vi "AprilTag Target Package Vers 2.vi"(0 "Camera Name":string="cam0") -> ()   [LabVIEW 2023]
uses:
  <vilib>/vision/Image Controls.llb/IMAQ Image.ctl
  <vilib>/Utility/config.llb/NI_LVConfig.lvlib
  <vilib>/Utility/config.llb/Write Key (String).vi
  Camera Set Up/Event Setup Types.ctl
  <vilib>/vision/NI_Vision_Development_Module.lvlib
  <vilib>/Rock Robotics/Network Tables/NT Write Numeric Array.vi
  <vilib>/Utility/config.llb/Read Key (String).vi
  <vilib>/vision/Pattern Matching.llb/IMAQ Match Range Setting.ctl
  <vilib>/vision/Shape Detection.llb/ShapeDetectionMatchOptions.ctl
  <vilib>/Rock Robotics/Network Tables/NT Write Integer Array.vi
panel:
  in  "Main":enum32{"Page 1", "Page 2"}(tab)
  out "Image":T1(plugin-control)
  in  "Settings":bool
  in  "Save":bool
  in  "Tools":bool
  out "Fps":dbl format="%#.0f"
  in  "Target Size":dbl=6.5
  out "Distance":dbl[](array[numeric]) format="%.1f"
  out "Angle":dbl[](array[numeric]) format="%.1f"
  in  "Find Tag Number":bool
  in  "Min Score":dbl=800.0
  in  "Min Rect Size (pix)":dbl
  in  "Max Rect Size (pix)":dbl
  in  "Home":bool
  in  "upper limit":sgl=1.2
  in  "lower limit":sgl=0.8
  # "Aspect Ratio"
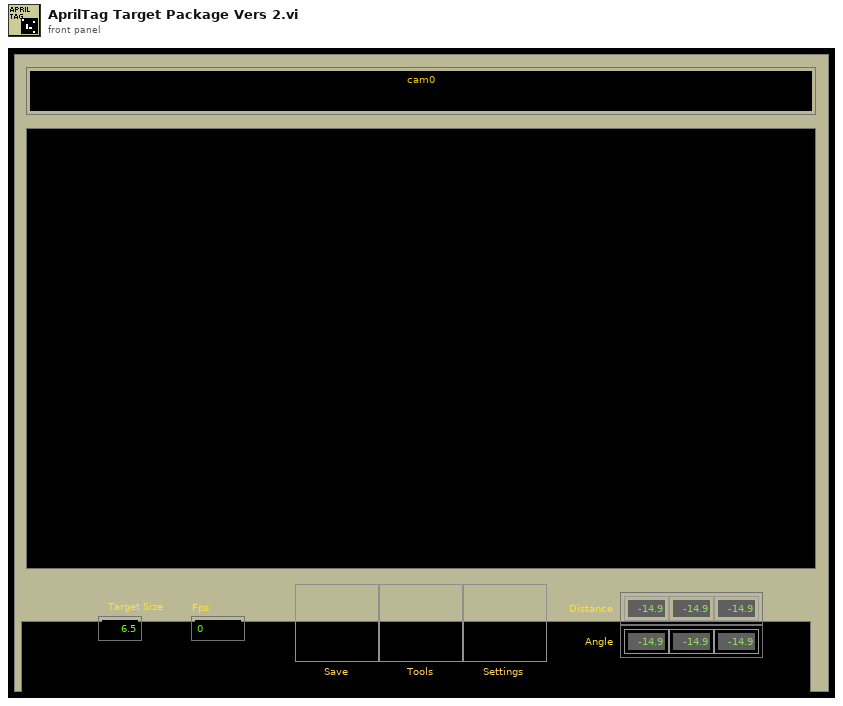
[diagram p1: front panel]
types:
  T1 = typedef "IMAQ Image.ctl" = refnum<image>
  T2 = typedef "Image Type" = u32
  T3 = typedef "ShapeDetectionMatchOptions.ctl" = cluster{"Rotation":bool, "Scale":bool, "Occlusion":bool, "Range Settings":T4[]}
  T4 = typedef "IMAQ Match Range Setting.ctl" = cluster{"Match Constraints":u32, "Min":dbl, "Max":dbl}
  T5 = cluster{"Min Width":dbl, "Max Width":dbl, "Min Height":dbl, "Max Height":dbl}
  T6 = typedef "Event Setup Types.ctl" = enum16{"Default", "Camera Loop Started", "Close Settings", "GreyScale", "Open Front Panel", "Save Data", "Exit"}
  T7 = cluster{"Corners":cluster{"X":sgl, "Y":sgl}[], "Angle":dbl, "Width":dbl, "Height":dbl, "Score":dbl}[]
  T8 = typedef "AprilTag Target Fields.ctl" = cluster{"diameter points":cluster{"first point":cluster{"x":dbl, "y":dbl}, "projected point":cluster{"x":dbl, "y":dbl}}, "normalized center":cluster{"x":dbl, "y":dbl}, "Overall Score":dbl, "Distance (ft)":dbl, "Offset Angle":dbl, "Tag corner points":cluster{"X":dbl, "Y":dbl}[], "Tag Center":cluster{"X":dbl, "Y":dbl}, "Tag Yaw":dbl, "Tag Pitch":dbl, "AprilTag Number":i32}
  T9 = typedef "Target Fields.ctl" = cluster{"diameter points":cluster{"first point":cluster{"x":dbl, "y":dbl}, "projected point":cluster{"x":dbl, "y":dbl}}, "normalized center":cluster{"x":dbl, "y":dbl}, "Overall Score":dbl, "Area Score":dbl, "Moment Score":dbl, "Aspect Score":dbl, "Distance (ft)":dbl, "Upper Goal":bool}
  T10 = typedef "NI_LVConfig.lvlib/Config Data RefNum.ctl" = refnum<k1>
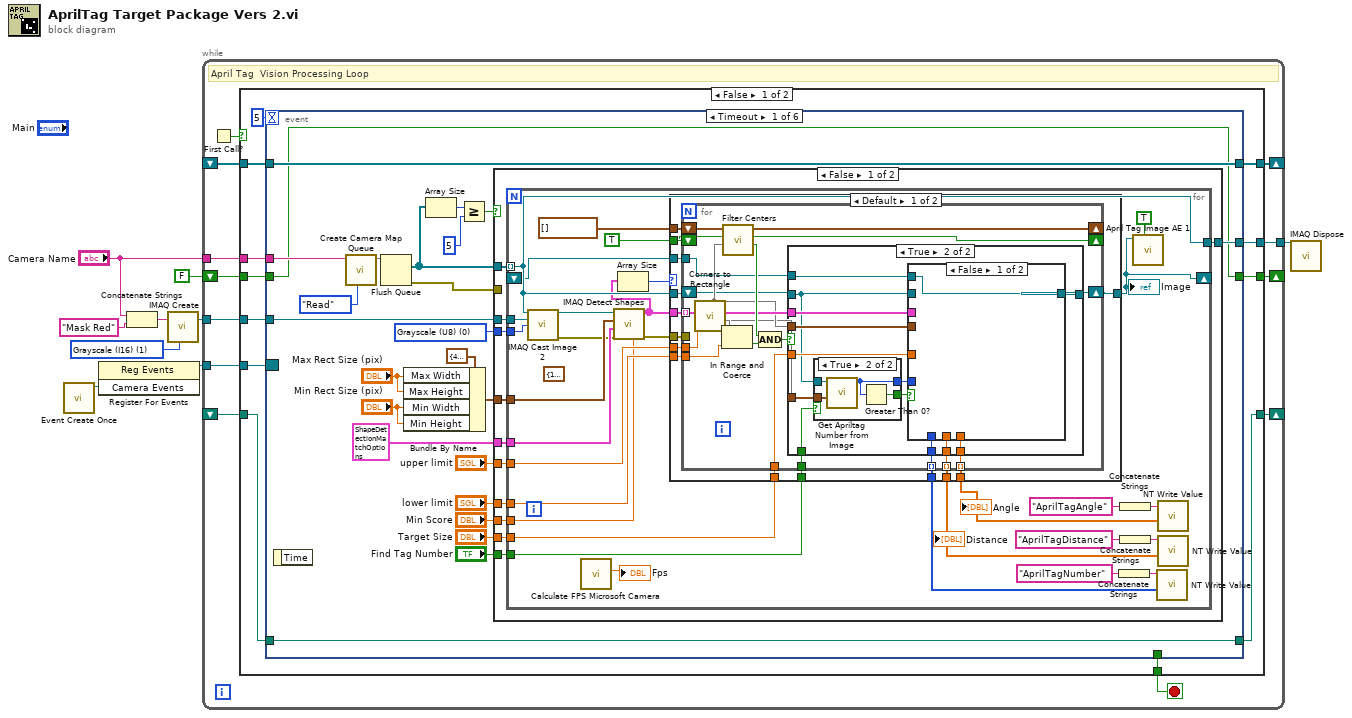
[diagram p0: block diagram]
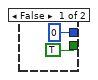
[diagram p3: hidden frame]
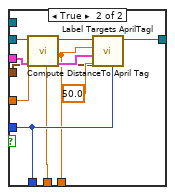
[diagram p4: hidden frame]
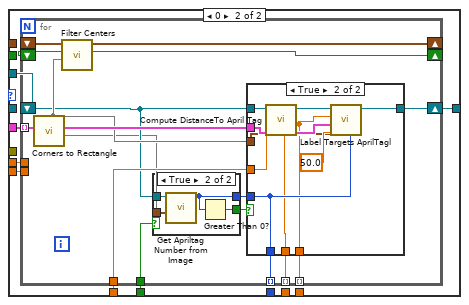
[diagram p5: hidden frame]
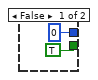
[diagram p6: hidden frame]
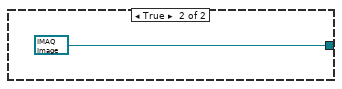
[diagram p8: hidden frame]
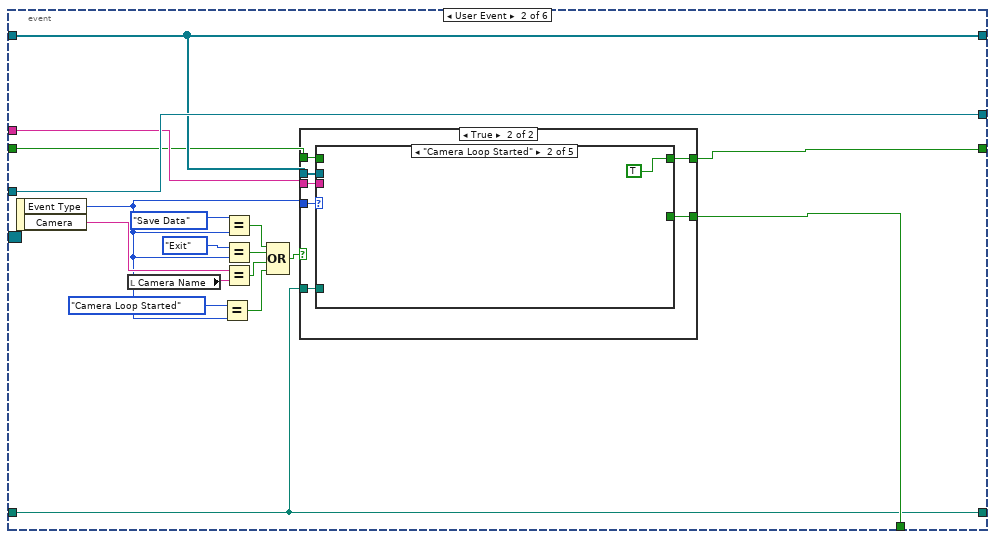
[diagram p9: hidden frame]
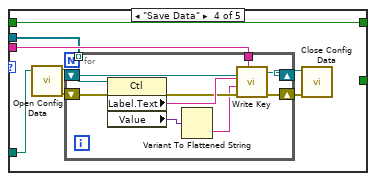
[diagram p13: hidden frame]
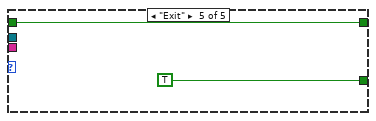
[diagram p14: hidden frame]
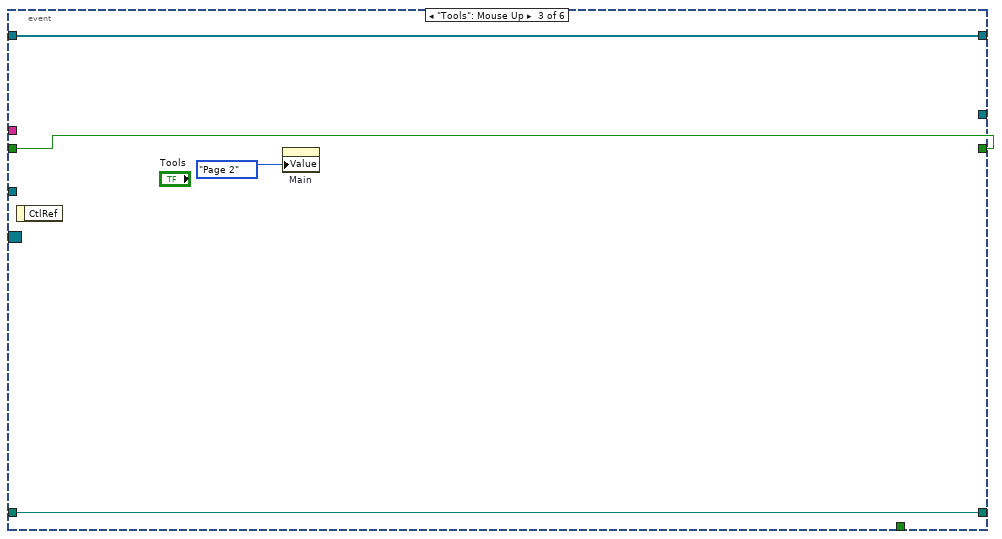
[diagram p15: hidden frame]
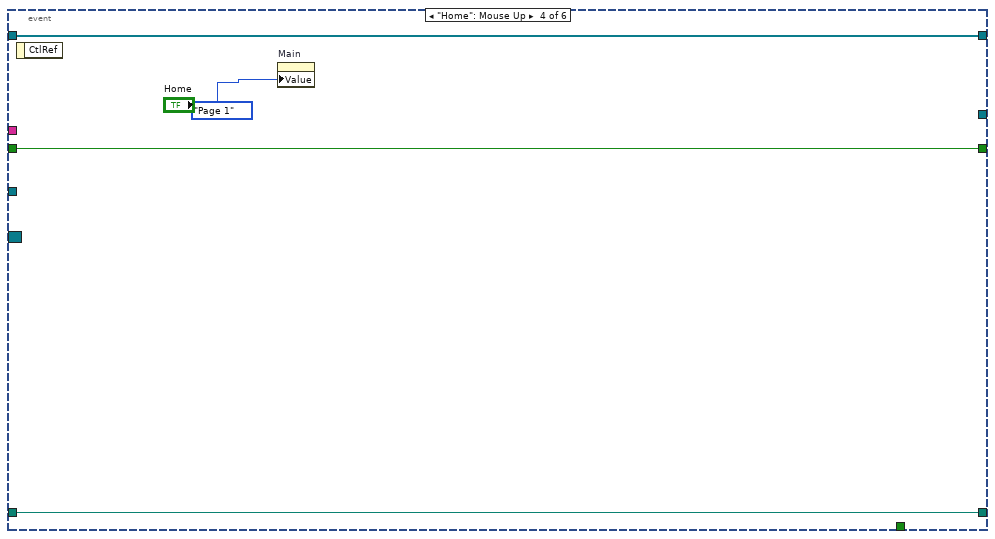
[diagram p16: hidden frame]
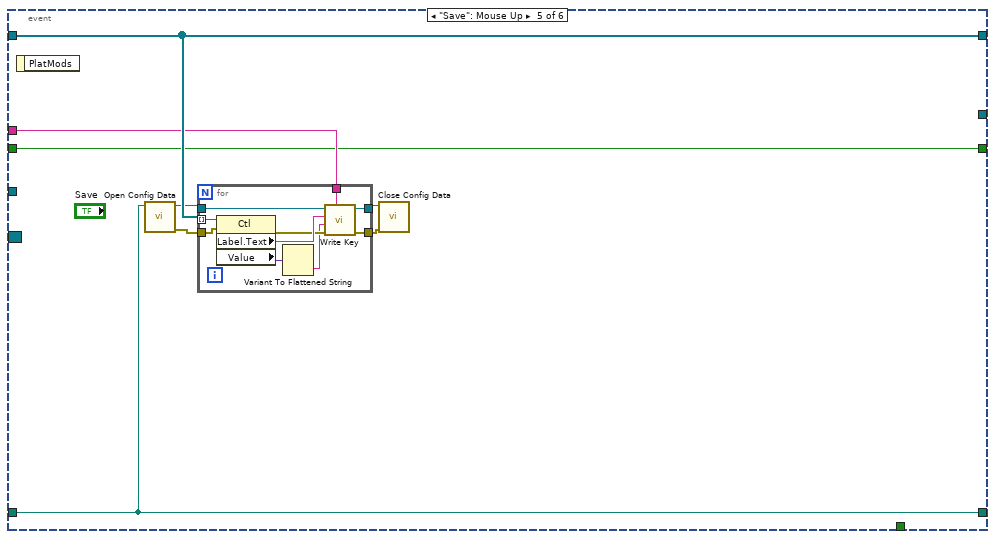
[diagram p17: hidden frame]
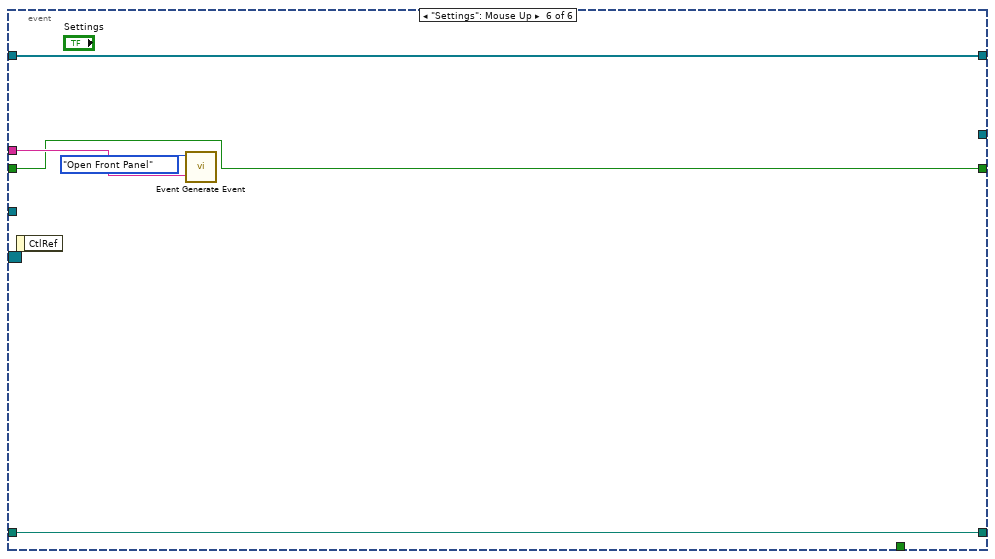
[diagram p18: hidden frame]
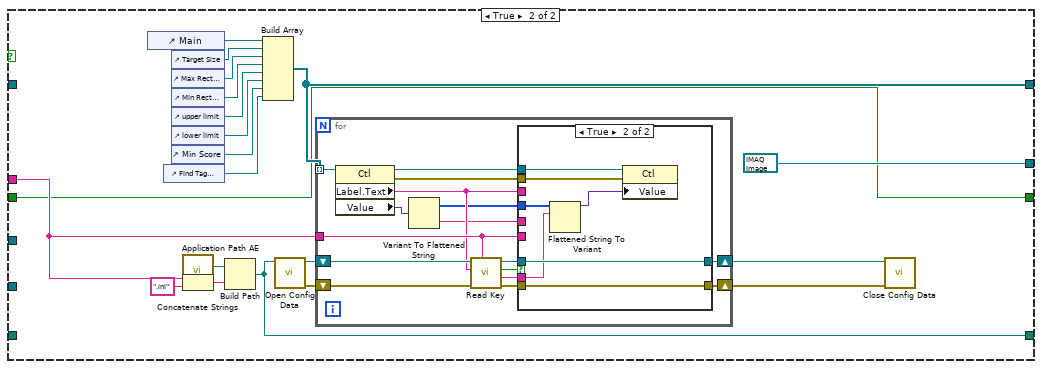
[diagram p19: hidden frame]
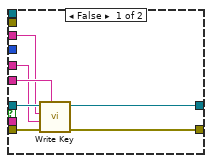
[diagram p20: hidden frame]
diagram:
  w6 = T2 1 items=["Grayscale (U8)", "Grayscale (I16)", "Grayscale (SGL)", "Complex (CSG)", "RGB (U32)", "HSL (U32)", "RGB (U64)", "Grayscale (U16)"] ("Image Type")
  n1 = call "Event Create Once.vi"() -> ("Camera Events"=w8:refnum<user-event>)  [unwired: 10 in, 1 out]
  n2 = register-events(w8) -> (reference out=w7:refnum<event-registration>)  [unwired: 2 in, 1 out]
  n3 = Concatenate Strings("Camera Name", "Mask Red" ("string")) -> (w5:string)
  n4 = call "IMAQ Create"("Image Name"=w5, "Image Type"=w6) -> ("New Image"=w9:T1)  [unwired: 2 in, 2 out]
  n5 = while {
    tunnel: w9 -> [w21]
    tunnel: [w20] -> w1
    tunnel: w7 -> [w19]
    tunnel: "Camera Name" -> [w17]
    shift-right: [w15] -> _
    shift-left: _ -> [w14]
    shift-right: [w13] -> _
    shift-left: _ -> [w12]
    shift-right: [w10] -> _
    shift-left: FALSE -> [w11]
    stop <- w18 stop-if-true
    # "April Tag  Vision Processing Loop"
    n6 = First Call?() -> (First Call?: T/F=w16:bool)
    n7 = case shown="False" w16 {
      tunnel: w21 -> [w33 _]
      tunnel: [w32 T1 refnum ("New Image")] -> w20
      tunnel: w19 -> [w31 _]
      tunnel: [w30 _] -> w18
      tunnel: w17 -> [w29 w303]
      tunnel: [w27 w299] -> w15
      tunnel: w14 -> [w28 _]
      tunnel: [w26 w302] -> w13
      tunnel: w12 -> [w24 _]
      tunnel: w11 -> [w23 w296]
      tunnel: [w22 w296] -> w10
      frame False {
        n8 = event shown="[0] Timeout" {
          selector: w31 -> [_ _ _ _ _ _]
          dyn-events: _ -> [_ _ _ _ _ _]
          timeout: 5 -> [_ _ _ _ _ _]
          tunnel: w33 -> [w56 w227 _ _ _ _]
          tunnel: [w57 w227 _ _ _ _] -> w32
          tunnel: [_ w226 _ _ _ _] -> w30
          tunnel: w29 -> [w53 w225 _ _ w270 w286]
          tunnel: w28 -> [w55 w223 w262 w266 w273 w289]
          tunnel: [w55 w223 w262 w266 w273 w289] -> w27
          tunnel: w24 -> [w54 w224 w261 w265 w274 w288]
          tunnel: [w54 w224 w261 w265 w274 w288] -> w26
          tunnel: w23 -> [w52 w214 w259 w263 w267 w285]
          tunnel: [w52 w213 w259 w263 w267 w285] -> w22
          event Timeout {
            w47 = T2 0 items=["Grayscale (U8)", "Grayscale (I16)", "Grayscale (SGL)", "Complex (CSG)", "RGB (U32)", "HSL (U32)", "RGB (U64)", "Grayscale (U16)"] ("Image Type")
            n9 = event-data() -> ()  [unwired: 1 in, 1 out]
            n10 = call "Create Camera Map Queue.vi"("Action"=enum16{"Read", "Write"}."Read", "Camera"=w53) -> (3:w49)  [unwired: 7 in, 2 out]
            n11 = Flush Queue(queue=w49) -> (remaining elements=w34:T1[], error out=w48:errorcluster)  [unwired: 1 in, 1 out]
            n12 = Bundle By Name(cluster=T5 {"Min Width"=40.0, "Max Width"=100.0, "Min Height"=40.0, "Max Height"=200.0} ("Rectangle Descriptor"), "Max Width"="Max Rect Size (pix)", "Max Height"="Max Rect Size (pix)", "Min Width"="Min Rect Size (pix)", "Min Height"="Min Rect Size (pix)") -> (w41:T5)
            n13 = Array Size(array=w34) -> (size(s)=w46:i32)
            n14 = Greater Or Equal?(x=w46, y=5) -> (x >= y?=w44:bool)
            n15 = case shown="False" w44 {
              tunnel: [w62 T1 refnum ("Image")] -> w57
              tunnel: w56 -> [w68 _]
              tunnel: "Target Size" -> [w67 _]
              tunnel: w34 -> [w66 _]
              tunnel: w48 -> [_ _]
              tunnel: w47 -> [w65 _]
              tunnel: w41 -> [w64 _]
              tunnel: T3 {"Rotation"=TRUE, "Scale"=TRUE, "Occlusion"=FALSE, "Range Settings"=[{"Match Constraints"=0, "Min"=-25.0, "Max"=25.0}, {"Match Constraints"=1, "Min"=25.0, "Max"=150.0}, {"Match Constraints"=0, "Min"=-25.0, "Max"=25.0}]} ("Match Options") -> [w63 _]
              tunnel: "lower limit" -> [w61 _]
              tunnel: "upper limit" -> [w60 _]
              tunnel: "Min Score" -> [w59 _]
              tunnel: "Find Tag Number" -> [w58 _]
              frame False {
                n16 = for {
                  tunnel: w68 -> [w98]
                  tunnel: w66 -> [w80] mode=indexing
                  tunnel: w67 -> [w91]
                  tunnel: w65 -> [w97]
                  tunnel: w64 -> [w95]
                  tunnel: w63 -> [w94]
                  tunnel: [w80] -> w62
                  tunnel: w61 -> [w89]
                  tunnel: w60 -> [w88]
                  tunnel: w59 -> [w79]
                  tunnel: w58 -> [w73]
                  shift-right: [w70] -> _
                  shift-left: _ -> [w69]
                  (unwired) cluster{"Lower value":sgl, "Upper value":sgl} {"Lower value"=128.0, "Upper value"=255.0} ("Range")
                  n17 = call "IMAQ Cast Image 2"("Image Src"=w80, "Image Dst"=w98, "Image Type"=w97) -> ("Image Dst Out"=w74:T1, "error out"=w78:errorcluster)  [unwired: 11 in]
                  n18 = call "Calculate FPS Microsoft Camera.vi"() -> ("Fps"=→"Fps":dbl)  [unwired: 11 in]
                  n19 = call-poly "IMAQ Detect Shapes"("Minimum match score"=w79, "error in (no error)"=w78, "Match Options"=w94, "Rectangle Descriptor"=w95, "Image"=w74) -> ("error out"=w90:errorcluster, "Rectangles"=w72:T7)  [unwired: 4 in, 1 out]
                  n20 = Array Size(array=w72) -> (size(s)=w71:i32)
                  n21 = case shown="Default" w71 {
                    tunnel: cluster{"X":dbl, "Y":dbl}[] [] ("Centers 2") -> [w112 _]
                    tunnel: TRUE -> [w111 _]
                    tunnel: w72 -> [w110 w173]
                    tunnel: w91 -> [w109 w172]
                    tunnel: w90 -> [w108 _]
                    tunnel: w89 -> [w107 w169]
                    tunnel: w88 -> [w106 w170]
                    tunnel: [w105 _] -> w84
                    tunnel: [w104 _] -> w82
                    tunnel: [w103 w168] -> w70
                    tunnel: w80 -> [w102 _]
                    tunnel: [w101 _] -> w75
                    tunnel: w73 -> [w100 w171]
                    tunnel: w69 -> [w99 w167]
                    frame Default {
                      n22 = for {
                        shift-right: [w120] -> w103
                        shift-left: w102 -> [w118]
                        shift-right: [w132] -> _
                        shift-left: w112 -> [w133]
                        shift-right: [w130] -> _
                        shift-left: w111 -> [w131]
                        tunnel: w110 -> [w116] mode=indexing
                        tunnel: w109 -> [w125]
                        tunnel: [w124] -> w104 mode=indexing
                        tunnel: [w123] -> w105 mode=indexing
                        tunnel: w108 -> [_]
                        tunnel: w107 -> [w122]
                        tunnel: w106 -> [w121]
                        tunnel: [w115] -> w101 mode=indexing
                        tunnel: w100 -> [w114]
                        tunnel: w99 -> [w113]
                        n23 = call "Corners to Rectangle.vi"("tag info"=w116) -> ("output cluster"=w126:T8, 4:w134, 5:w119, 6:w117)  [unwired: 7 in]
                        n24 = In Range and Coerce(upper limit=w121, x=w134, lower limit=w122) -> (In Range?=w128:bool)  [unwired: 1 out]
                        n25 = call "Filter Centers.vi"("Center"=w119, "First time"=w131, "Centers"=w133) -> ("Added"=w129:bool, "First time Out"=w130:bool, "Centers 2"=w132:cluster{"X":dbl, "Y":dbl}[])  [unwired: 6 in]
                        n26 = Compound Arithmetic op=AND(w129, w128) -> (w127:bool)
                        n27 = case shown="True" w127 {
                          tunnel: w118 -> [_ w141]
                          tunnel: [w135 w148] -> w120
                          tunnel: w126 -> [_ w147]
                          tunnel: w125 -> [_ w146]
                          tunnel: [_ w145] -> w124
                          tunnel: [_ w144] -> w123
                          tunnel: w119 -> [_ w143]
                          tunnel: w117 -> [_ w142]
                          tunnel: [_ w139] -> w115
                          tunnel: w114 -> [_ w137]
                          tunnel: w113 -> [w135 w136]
                          frame False {
                          }
                          frame True {
                            n28 = case shown="True" w137 {
                              tunnel: w142 -> [_ w154]
                              tunnel: w141 -> [_ w153]
                              tunnel: [0 ("AprilTag#") w152] -> w140
                              tunnel: [TRUE w151] -> w138
                              frame False {
                              }
                              frame True {
                                n29 = call "Get Apriltag Number from Image.vi"("Corners"=w154, "Image"=w153) -> ("AprilTag#"=w152:i32)  [unwired: 9 in]
                                n30 = Greater Than 0?(x=w152) -> (x > 0?=w151:bool)
                              }
                            }
                            n31 = case shown="False" w138 {
                              tunnel: [w155 w166] -> w148
                              tunnel: w147 -> [_ w163]
                              tunnel: w146 -> [_ w162]
                              tunnel: [_ w156] -> w145
                              tunnel: [_ w157] -> w144
                              tunnel: w143 -> [_ w160]
                              tunnel: w141 -> [_ w159]
                              tunnel: w140 -> [_ w158]
                              tunnel: [_ w158] -> w139
                              tunnel: w136 -> [w155 _]
                              frame False {
                              }
                              frame True {
                                n32 = call "Compute DistanceTo April Tag.vi"("Target Width (in)"=w162, "results"=w163, "Image Src"=w159) -> ("results out"=w164:T9, "Off Angle"=w157:dbl, "Image Dst Out"=w161:T1, "Distance"=w156:dbl)  [unwired: 4 in, 1 out]
                                n33 = call "Label Targets AprilTagl.vi"(4:w158, 6:w160, 8:50.0 ("Score Threshold"), "results"=w164, "Angle"=w157, "Image in"=w161) -> ("Image out"=w166:T1)  [unwired: 5 in]
                              }
                            }
                          }
                        }
                      }
                    }
                    frame 0 {
                      n34 = for {
                        shift-right: [w182] -> w168
                        shift-left: w167 -> [w180]
                        shift-right: [w189] -> _
                        shift-left: _ -> [w190]
                        shift-right: [w187] -> _
                        shift-left: _ -> [w188]
                        tunnel: w173 -> [w178] mode=indexing
                        tunnel: w172 -> [w185]
                        tunnel: [w184] -> _ mode=indexing
                        tunnel: [w183] -> _ mode=indexing
                        tunnel: w169 -> [_]
                        tunnel: w170 -> [_]
                        tunnel: [w177] -> _ mode=indexing
                        tunnel: w171 -> [w176]
                        n35 = call "Corners to Rectangle.vi"("tag info"=w178) -> ("output cluster"=w186:T8, 5:w181, 6:w179)  [unwired: 8 in]
                        n36 = call "Filter Centers.vi"("Center"=w181, "First time"=w188, "Centers"=w190) -> ("First time Out"=w187:bool, "Centers 2"=w189:cluster{"X":dbl, "Y":dbl}[])  [unwired: 6 in, 1 out]
                        n37 = case shown="True" w176 {
                          tunnel: w179 -> [_ w196]
                          tunnel: w180 -> [_ w195]
                          tunnel: [0 ("AprilTag#") w194] -> w175
                          tunnel: [TRUE w193] -> w174
                          frame False {
                          }
                          frame True {
                            n38 = call "Get Apriltag Number from Image.vi"("Corners"=w196, "Image"=w195) -> ("AprilTag#"=w194:i32)  [unwired: 9 in]
                            n39 = Greater Than 0?(x=w194) -> (x > 0?=w193:bool)
                          }
                        }
                        n40 = case shown="True" w174 {
                          tunnel: [w197 w208] -> w182
                          tunnel: w186 -> [_ w205]
                          tunnel: w185 -> [_ w204]
                          tunnel: [_ w198] -> w184
                          tunnel: [_ w199] -> w183
                          tunnel: w181 -> [_ w202]
                          tunnel: w180 -> [w197 w201]
                          tunnel: w175 -> [_ w200]
                          tunnel: [_ w200] -> w177
                          frame False {
                          }
                          frame True {
                            n41 = call "Compute DistanceTo April Tag.vi"("Target Width (in)"=w204, "results"=w205, "Image Src"=w201) -> ("results out"=w206:T9, "Off Angle"=w199:dbl, "Image Dst Out"=w203:T1, "Distance"=w198:dbl)  [unwired: 4 in, 1 out]
                            n42 = call "Label Targets AprilTagl.vi"(4:w200, 6:w202, 8:50.0 ("Score Threshold"), "results"=w206, "Angle"=w199, "Image in"=w203) -> ("Image out"=w208:T1)  [unwired: 5 in]
                          }
                        }
                      }
                    }
                  }
                  "Image" <- w70
                  "Angle" <- w84
                  "Distance" <- w82
                  n43 = Concatenate Strings("AprilTagNumber" ("Name")) -> (w76:string)
                  n44 = Concatenate Strings("AprilTagAngle" ("Name")) -> (w83:string)
                  n45 = Concatenate Strings("AprilTagDistance" ("Name")) -> (w87:string)
                  n46 = call "April Tag Image AE 1.vi"("Update"=TRUE, "Ball Image in"=w70) -> ()  [unwired: 9 in, 1 out]
                  n47 = call-poly <vilib>:"NT Write Value.vi"("value"=w75, "name"=w76) -> ()  [unwired: 9 in, 1 out]
                  n48 = call-poly <vilib>:"NT Write Value.vi"("value"=w84, "name"=w83) -> ()  [unwired: 9 in, 1 out]
                  n49 = call-poly <vilib>:"NT Write Value.vi"("value"=w82, "name"=w87) -> ()  [unwired: 9 in, 1 out]
                }
              }
              frame True {
              }
            }
          }
          event User Event {
            n50 = event-data() -> ("Event Type"=w212:T6, "Camera"=w217:string)  [unwired: 1 in]
            n51 = local read "Camera Name"() -> (w218:string)
            n52 = Equal?(x=Event_Setup_Types."Camera Loop Started", y=w212) -> (x = y?=w210:bool)
            n53 = Equal?(x=Event_Setup_Types."Save Data", y=w212) -> (x = y?=w219:bool)
            n54 = Equal?(x=Event_Setup_Types."Exit", y=w212) -> (x = y?=w221:bool)
            n55 = Equal?(x=w217, y=w218) -> (x = y?=w216:bool)
            n56 = Compound Arithmetic op=OR(w219, w221, w216, w210) -> (w215:bool)
            n57 = case shown="True" w215 {
              tunnel: w212 -> [_ w235]
              tunnel: [_ w234] -> w226
              tunnel: w225 -> [_ w233]
              tunnel: w224 -> [_ w232]
              tunnel: w223 -> [_ w231]
              tunnel: w214 -> [w228 w230]
              tunnel: [w228 w229] -> w213
              frame False {
              }
              frame True {
                n58 = case shown="\"Camera Loop Started\"" w235 {
                  tunnel: [_ _ _ _ TRUE] -> w234
                  tunnel: w233 -> [_ _ _ w242 _]
                  tunnel: w232 -> [_ _ _ w241 _]
                  tunnel: w231 -> [_ _ _ w240 _]
                  tunnel: w230 -> [w236 _ w238 w239 w257]
                  tunnel: [w236 TRUE w238 w239 w257] -> w229
                  frame "Default" {
                  }
                  frame "Camera Loop Started" {
                  }
                  frame "Open Front Panel" {
                  }
                  frame "Save Data" {
                    n59 = call <vilib>:"Open Config Data.vi"("configuration file path"=w241) -> ("error out"=w243:errorcluster, "refnum"=w246:T10)  [unwired: 8 in, 1 out]
                    n60 = for {
                      tunnel: w242 -> [w252]
                      tunnel: w240 -> [w251] mode=indexing
                      shift-right: [w255] -> w245
                      shift-left: w246 -> [w256]
                      shift-right: [w254] -> w244
                      shift-left: w243 -> [w253]
                      n61 = property class="Ctl"(reference=w251, error in=w253) -> (error out=w248:errorcluster, "Label.Text"=w250:string, "Value"=w249:variant)  [unwired: 1 out]
                      n62 = Variant To Flattened String(Variant=w249) -> (data string=w247:string)  [unwired: 1 out]
                      n63 = call-poly <vilib>:"Write Key.vi"("section"=w252, "error in (no error)"=w248, "value"=w247, "key"=w250, "refnum"=w256) -> ("error out"=w254:errorcluster, "refnum out"=w255:T10)  [unwired: 4 in, 1 out]
                    }
                    n64 = call <vilib>:"Close Config Data.vi"("error in (no error)"=w244, "refnum"=w245) -> ()  [unwired: 8 in, 2 out]
                  }
                  frame "Exit" {
                  }
                }
              }
            }
          }
          event "Tools": Mouse Up {
            n65 = event-data() -> ()  [unwired: 1 in, 1 out]
            n66 = property on="Main" class="TabCtl (strict)"("Value"=enum32{"Page 1", "Page 2"}."Page 2" ("Main")) -> ()  [unwired: 2 in, 2 out]
          }
          event "Home": Mouse Up {
            n67 = event-data() -> ()  [unwired: 1 in, 1 out]
            n68 = property on="Main" class="TabCtl (strict)"("Value"=enum32{"Page 1", "Page 2"}."Page 1" ("Main")) -> ()  [unwired: 2 in, 2 out]
          }
          event "Save": Mouse Up {
            n69 = event-data() -> ()  [unwired: 1 in, 1 out]
            n70 = call <vilib>:"Open Config Data.vi"("configuration file path"=w274) -> ("error out"=w271:errorcluster, "refnum"=w272:T10)  [unwired: 8 in, 1 out]
            n71 = for {
              tunnel: w273 -> [w284] mode=indexing
              tunnel: w272 -> [w283]
              tunnel: w271 -> [w282]
              tunnel: w270 -> [w278]
              tunnel: [w276] -> w269
              tunnel: [w275] -> w268
              n72 = property class="Ctl"(reference=w284, error in=w282) -> (error out=w279:errorcluster, "Label.Text"=w281:string, "Value"=w280:variant)  [unwired: 1 out]
              n73 = Variant To Flattened String(Variant=w280) -> (data string=w277:string)  [unwired: 1 out]
              n74 = call-poly <vilib>:"Write Key.vi"("section"=w278, "error in (no error)"=w279, "value"=w277, "key"=w281, "refnum"=w283) -> ("error out"=w276:errorcluster, "refnum out"=w275:T10)  [unwired: 4 in, 1 out]
            }
            n75 = call <vilib>:"Close Config Data.vi"("error in (no error)"=w269, "refnum"=w268) -> ()  [unwired: 8 in, 2 out]
          }
          event "Settings": Mouse Up {
            n76 = event-data() -> ()  [unwired: 1 in, 1 out]
            n77 = call "Event Generate Event.vi"("Camera Name"=w286, "Event Type"=Event_Setup_Types."Open Front Panel") -> ()  [unwired: 10 in]
          }
        }
      }
      frame True {
        n78 = control-ref of="Main"() -> (w298:refnum<vi>)
        n79 = control-ref of="Find Tag Number"() -> (w290:refnum<vi>)
        n80 = control-ref of="Target Size"() -> (w297:refnum<vi>)
        n81 = control-ref of="Max Rect Size (pix)"() -> (w295:refnum<vi>)
        n82 = control-ref of="Min Rect Size (pix)"() -> (w294:refnum<vi>)
        n83 = control-ref of="upper limit"() -> (w293:refnum<vi>)
        n84 = control-ref of="lower limit"() -> (w292:refnum<vi>)
        n85 = control-ref of="Min Score"() -> (w291:refnum<vi>)
        n86 = call "Application Path AE.vi"() -> ("Application Path out"=w300:path)  [unwired: 11 in]
        n87 = Concatenate Strings(w303, ".ini" ("name or relative path")) -> (w308:string)
        n88 = Build Path(base path=w300, name or relative path=w308) -> (appended path=w302:path)
        n89 = Build Array(w298, w297, w295, w294, w293, w292, w291, w290) -> (w299:refnum<vi>[])
        n90 = call <vilib>:"Open Config Data.vi"("configuration file path"=w302) -> ("error out"=w301:errorcluster, "refnum"=w307:T10)  [unwired: 8 in, 1 out]
        n91 = for {
          tunnel: w303 -> [w322]
          tunnel: w299 -> [w312] mode=indexing
          shift-right: [w324] -> w306
          shift-left: w307 -> [w325]
          shift-right: [w323] -> w305
          shift-left: w301 -> [w321]
          n92 = property class="Ctl"(reference=w312) -> (reference out=w318:refnum<vi>, error out=w317:errorcluster, "Label.Text"=w315:string, "Value"=w311:variant)  [unwired: 1 in]
          n93 = Variant To Flattened String(Variant=w311) -> (data string=w313:string, 1:w310:i16[])
          n94 = call-poly <vilib>:"Read Key.vi"("section"=w322, "error in (no error)"=w321, "key"=w315, "refnum"=w325) -> ("error out"=w314:errorcluster, "value"=w319:string, "found?"=w320:bool, "refnum out"=w316:T10)  [unwired: 4 in]
          n95 = case shown="True" w320 {
            tunnel: w319 -> [_ w334]
            tunnel: w318 -> [_ w339]
            tunnel: w317 -> [_ w338]
            tunnel: w316 -> [w332 w337]
            tunnel: w322 -> [w331 _]
            tunnel: w315 -> [w330 _]
            tunnel: [w329 w337] -> w324
            tunnel: w314 -> [w328 w336]
            tunnel: [w327 w336] -> w323
            tunnel: w313 -> [w326 _]
            tunnel: w310 -> [_ w333]
            frame False {
              n96 = call-poly <vilib>:"Write Key.vi"("section"=w331, "error in (no error)"=w328, "value"=w326, "key"=w330, "refnum"=w332) -> ("error out"=w327:errorcluster, "refnum out"=w329:T10)  [unwired: 4 in, 1 out]
            }
            frame True {
              n97 = Flattened String To Variant(6:w334, 7:w333) -> (3:w335:variant)  [unwired: 1 in, 1 out]
              n98 = property class="Ctl"(reference=w339, error in=w338, "Value"=w335) -> ()  [unwired: 2 out]
            }
          }
        }
        n99 = call <vilib>:"Close Config Data.vi"("error in (no error)"=w305, "refnum"=w306) -> ()  [unwired: 8 in, 2 out]
      }
    }
  }
  n100 = call "IMAQ Dispose"("Image"=w1) -> ()  [unwired: 5 in, 1 out]
